vi "Move stage to diode position.vi"(8 "error in (no error) 3":errorcluster) -> (0 "error out":errorcluster)   [LabVIEW 2016]
uses:
  <vilib>/Utility/file.llb/Read From Spreadsheet File (string).vi
panel:
  out "Y":string
  out "X":string
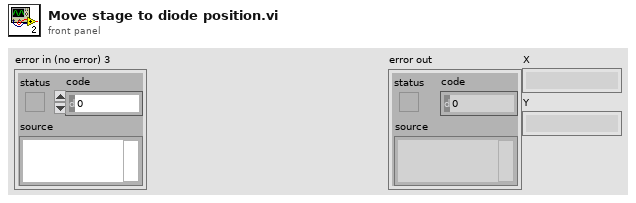
[diagram p1: front panel]
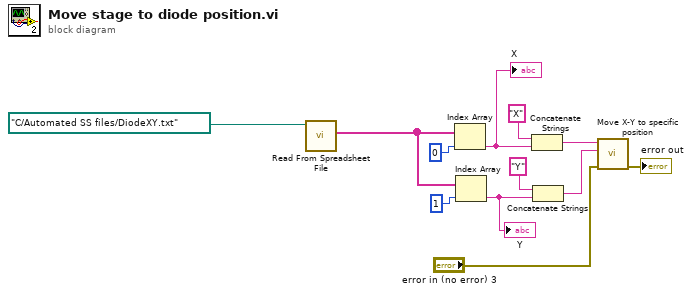
[diagram p0: block diagram]
diagram:
  n1 = call-poly <vilib>:"Read From Spreadsheet File.vi"("file path (dialog if empty)"=path "C:/Automated SS files/DiodeXY.txt") -> ("first row"=w5:string[])  [unwired: 6 in, 4 out]
  n2 = Index Array(array=w5, index=0) -> (element=w6:string)
  "X" <- w6
  n3 = Index Array(array=w5, index=1) -> (element=w7:string)
  "Y" <- w7
  n4 = Concatenate Strings("X", w6) -> (w10:string)
  n5 = Concatenate Strings("Y", w7) -> (w11:string)
  n6 = call "Move X-Y to specific position.vi"("error in (no error) 3"="error in (no error) 3", "position 2"=w11, "position 1"=w10) -> ("error out 3"=→"error out":errorcluster)  [unwired: 4 in, 4 out]
